vi "Apply Event Value.vi"(0 "Tosca in":refnum<class "Parameters.lvclass">, 5 "Event":string, 7 "Criterion":string, 9 "Value":dbl, 11 "error in (no error)":errorcluster) -> (4 "Tosca out":refnum<class "Parameters.lvclass">, 15 "error out":errorcluster)   [LabVIEW 2015, in "Parameters.lvclass"]
uses:
  Parameters.lvclass
  Parameters.lvclass/Parameters.ctl
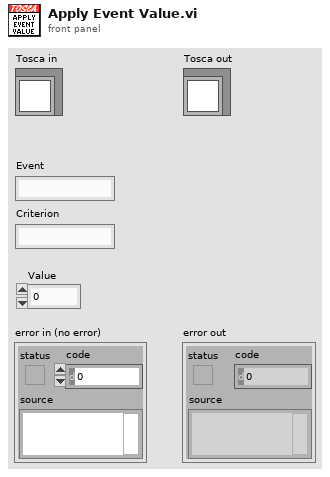
[diagram p1: front panel]
types:
  T1 = typedef "Tosca-Input Event.ctl" = cluster{"Name":string, "Criteria":T2[], "Operators":enum16{"AND", "OR"}[], "Accumulator":T4}
  T2 = typedef "Tosca-Input Criterion.ctl" = cluster{"DigInput":i32, "State":T3, "Time (ms)":i32, "Name":string}
  T3 = typedef "Logic State.ctl" = enum16{"Low", "High", "Rising", "Falling"}
  T4 = typedef "Tosca-Accumulator.ctl" = cluster{"active":bool, "N":i32, "T":dbl, "Imax":dbl, "latency":dbl}
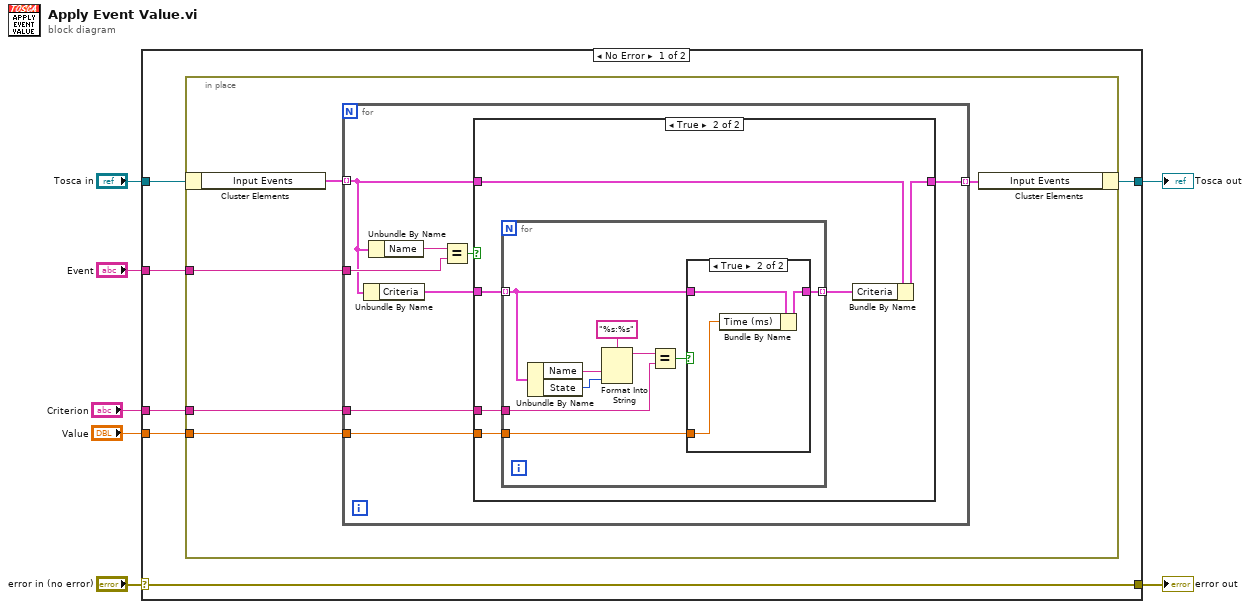
[diagram p0: block diagram]
diagram:
  n1 = case shown="No Error" "error in (no error)" {
    selector: "error in (no error)" -> [w13 w48]
    tunnel: [w13 w48] -> w6
    tunnel: [w10 w47] -> w4
    tunnel: "Tosca in" -> [w12 w47]
    tunnel: "Event" -> [w11 _]
    tunnel: "Criterion" -> [w9 _]
    tunnel: "Value" -> [w8 _]
    frame No Error {
      n2 = in-place {
        in-place-border: w11 -> [w17]
        in-place-border: w9 -> [w15]
        in-place-border: w8 -> [w14]
        n3 = in-place-cluster #1(w12) -> ("Input Events"=w18:T1[])
        n4 = for {
          tunnel: w18 -> [w22] mode=indexing
          tunnel: w17 -> [w25]
          tunnel: [w21] -> w16 mode=indexing
          tunnel: w15 -> [w20]
          tunnel: w14 -> [w19]
          n5 = Unbundle By Name(w22) -> ("Criteria"=w23:T2[])
          n6 = Unbundle By Name(w22) -> ("Name"=w26:string)
          n7 = Equal?(x=w26, y=w25) -> (x = y?=w24:bool)
          n8 = case shown="True" w24 {
            tunnel: w23 -> [_ w33]
            tunnel: w22 -> [w27 w30]
            tunnel: [w27 w28] -> w21
            tunnel: w20 -> [_ w32]
            tunnel: w19 -> [_ w31]
            frame False {
            }
            frame True {
              n9 = for {
                tunnel: w33 -> [w37] mode=indexing
                tunnel: w32 -> [w38]
                tunnel: w31 -> [w35]
                tunnel: [w34] -> w29 mode=indexing
                n10 = Unbundle By Name(w37) -> ("Name"=w41:string, "State"=w40:T3)
                n11 = Format Into String(format string="%s:%s", w41, w40) -> (resulting string=w39:string)  [unwired: 2 in, 1 out]
                n12 = Equal?(x=w39, y=w38) -> (x = y?=w36:bool)
                n13 = case shown="True" w36 {
                  tunnel: w37 -> [w43 w46]
                  tunnel: w35 -> [_ w45]
                  tunnel: [w43 w44] -> w34
                  frame False {
                  }
                  frame True {
                    n14 = Bundle By Name(cluster=w46, "Time (ms)"=w45) -> (w44:T2)
                  }
                }
              }
              n15 = Bundle By Name(cluster=w30, "Criteria"=w29) -> (w28:T1)
            }
          }
        }
        n16 = in-place-cluster #1("Input Events"=w16) -> (w10:refnum<class "Parameters.lvclass">)
      }
    }
    frame Error {
    }
  }
  "error out" <- w6
  "Tosca out" <- w4
